vi "PYTHON Set Integer Data__ogtk.vi"(4 "error in (no error)":errorcluster, 5 "value":i32, 6 "variable name":string, 7 "Python Session in":T1) -> (0 "error out":errorcluster, 3 "Python Session out":T1)   [LabVIEW 2014]
uses:
  <userlib>/_OpenG.lib/labpython/labpython.llb/PYTHON Session Refnum__ogtk.ctl
  <userlib>/_OpenG.lib/labpython/lvpython.dll
panel:
  # "PYTHON Set Integer Data.vi\n\nSet the value of an integer variable in the session context\n\nCopyright (C) 2002 Rolf Kalbermatter rolf.kalbermatter@citeng.com\nCopyright (C) 2002 James Kring jim@jimkring.com\n\nPlease visit http://www.OpenG.org to learn about the\nOpen Source LabVIEW software movement.\n\nThis library is free software; you can redistribute it and/or\nmodify it under the terms of the GNU Lesser General Public\nLicense as published by the Free Software Foundation; either\nversion 2.1 of the License, or (at your option) any later version.\nThis library is distributed in the hope that it will be useful,\nbut WITHOUT ANY WARRANTY; without even the implied warranty of\nMERCHANTABILITY or FITNESS FOR A PARTICULAR PURPOSE. See the GNU\nLesser General Public License for more details.\nYou should have received a copy of the GNU Lesser General Public\nLicense along with this library; if not, write to the Free Software\nFoundation, Inc., 59 Temple Place, Suite 330, Boston, MA 02111-1307 USA"
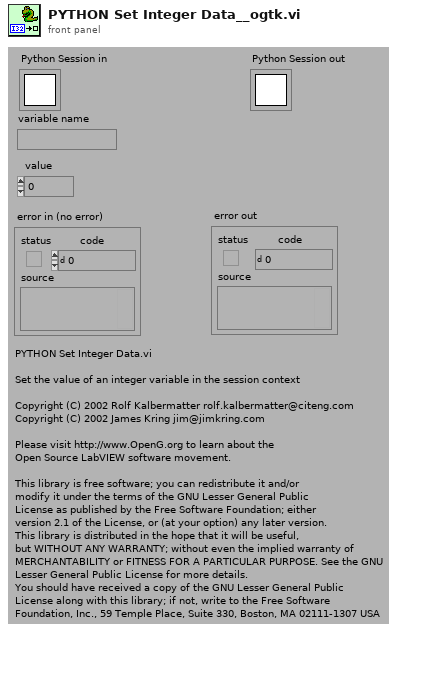
[diagram p1: front panel]
types:
  T1 = typedef "PYTHON Session Refnum__ogtk.ctl" = refnum<k1>
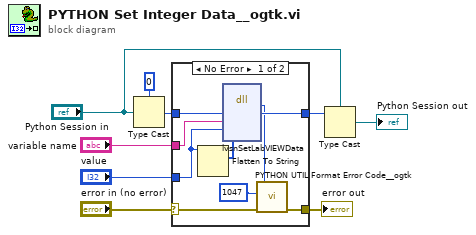
[diagram p0: block diagram]
diagram:
  n1 = Type Cast(type=u32 0 ("session"), x="Python Session in") -> (*(type *) &x=w2:u32)
  n2 = case shown="No Error" "error in (no error)" {
    selector: "error in (no error)" -> [w14 w20]
    tunnel: [w16 w19] -> w1
    tunnel: [w12 w20] -> w8
    tunnel: w2 -> [w18 w19]
    tunnel: "variable name" -> [w17 _]
    tunnel: "value" -> [w10 _]
    frame No Error {
      n3 = Flatten To String(anything=w10) -> (type string=w11:i16[])  [unwired: 3 in, 2 out]
      n4 = dll-call lib="C:/Program Files (x86)/National Instruments/LabVIEW 2014/user.lib/_OpenG.lib/labpython/lvpython.*" fn="lvsnSetLabVIEWData"("session"=w18, "name"=w17, "value"=w10, "type"=w11) -> (w15:i32, "session"=w16:u32)  [unwired: 6 in, 2 out]
      n5 = call <userlib>:"PYTHON UTIL Format Error Code__ogtk.vi"("error in (no error)"=w14, "code"=1047, "Bool32"=w15) -> ("error out"=w12:errorcluster)  [unwired: 4 in]
    }
    frame Error {
    }
  }
  "error out" <- w8
  n6 = Type Cast(type="Python Session in", x=w1) -> (*(type *) &x=→"Python Session out":T1)
